vi "Write Measurement Times.vi"(8 "error in (no error)":errorcluster, 10 "Measurement Times":string[](array[string]), 11 "ModeSwitch Eval in":refnum<class "ModeSwitch Eval.lvclass">) -> (0 "error out":errorcluster, 3 "ModeSwitch Eval out":refnum<class "ModeSwitch Eval.lvclass">)   [LabVIEW 2016, in "SeqAuto Evaluations.lvlib" / "ModeSwitch Eval.lvclass"]
uses:
  ModeSwitch Eval.lvclass
  ModeSwitch Eval.lvclass/ModeSwitch Eval.ctl
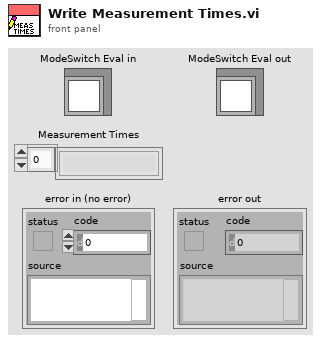
[diagram p1: front panel]
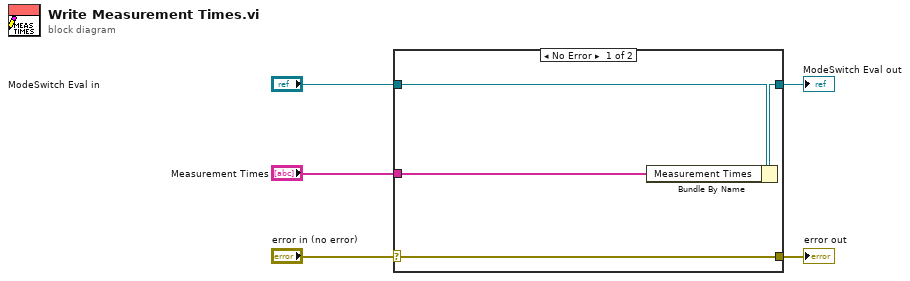
[diagram p0: block diagram]
diagram:
  n1 = case shown="No Error" "error in (no error)" {
    selector: "error in (no error)" -> [w9 w10]
    tunnel: [w9 w10] -> w4
    tunnel: [w7 w11] -> w2
    tunnel: "ModeSwitch Eval in" -> [w8 w11]
    tunnel: "Measurement Times" -> [w6 _]
    frame No Error {
      n2 = Bundle By Name(cluster=w8, "Measurement Times"=w6) -> (w7:refnum<class "ModeSwitch Eval.lvclass">)
    }
    frame Error {
    }
  }
  "error out" <- w4
  "ModeSwitch Eval out" <- w2
